vi "getRange.vi"(8 "error in (no error)":errorcluster, 11 "DmmNiPxi in":refnum<class "DmmNi.lvclass">) -> (0 "error out":errorcluster, 2 "range":dbl, 3 "DmmNiPxi out":refnum<class "DmmNi.lvclass">)   [LabVIEW 2023, in "DmmNi.lvclass"]
doc: "<b>Author:</b> Wolfgang\n<b>Description:</b> return measurement range of the dmm based for the actual selected mode"
uses:
  DmmNi.lvclass
  DmmNi.lvclass/DmmNi.ctl
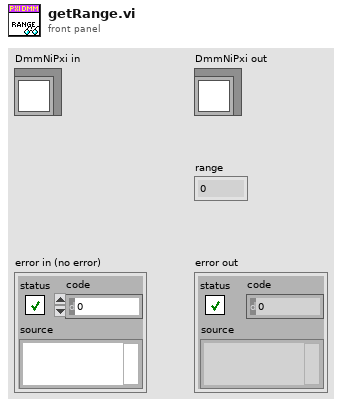
[diagram p1: front panel]
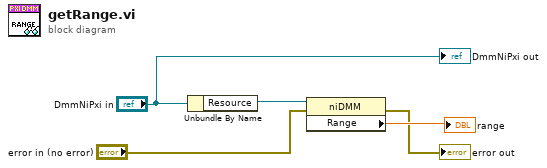
[diagram p0: block diagram]
diagram:
  n1 = Unbundle By Name("DmmNiPxi in") -> ("Resource"=w5:refnum<k15>)
  n2 = property class="niDMM"(reference=w5, error in="error in (no error)") -> (error out=→"error out":errorcluster, "Range"=→"range":dbl)  [unwired: 1 out]
  "DmmNiPxi out" <- "DmmNiPxi in"
